vi "Receive Shortcut Menu Selection Event.vi"(8 "error in (no error)":errorcluster, 10 "ShortcutMenuSelectionMsg":refnum<class "ShortcutMenuSelectionMsg.lvclass">, 11 "File Explorer In":refnum<class "File Explorer.lvclass">) -> (0 "error out":errorcluster, 3 "File Explorer Out":refnum<class "File Explorer.lvclass">)   [LabVIEW 2020, in "File Explorer.lvlib" / "File Explorer.lvclass"]
doc: "<License>\nCopyright © 2017 Composed Systems, LLC | All rights reserved\nwww.composed.io\n\nAuthor: Ethan Stern <ethan.stern@composed.io>\n\nThis software is provided \"AS IS\" WITHOUT WARRANTIES, either express or implied, AND IS FOR EDUCATIONAL PURPOSES ONLY.\n</License>"
uses:
  <vilib>/gpm_packages/@cs/file-explorer-extension/Source/File Explorer/File Explorer/File Explorer.lvclass
  <vilib>/gpm_packages/@cs/mva-viewable/Source/ActorEvents/IEventAggregator Messages/ShortcutMenuSelectionMsg/ShortcutMenuSelectionMsg.lvclass
  <vilib>/gpm_packages/@cs/mva-viewable/Source/ActorEvents/IEventAggregator Messages/ShortcutMenuSelectionMsg/ShortcutMenuSelectionMsg.lvclass/ShortcutMenuSelectionMsg.ctl
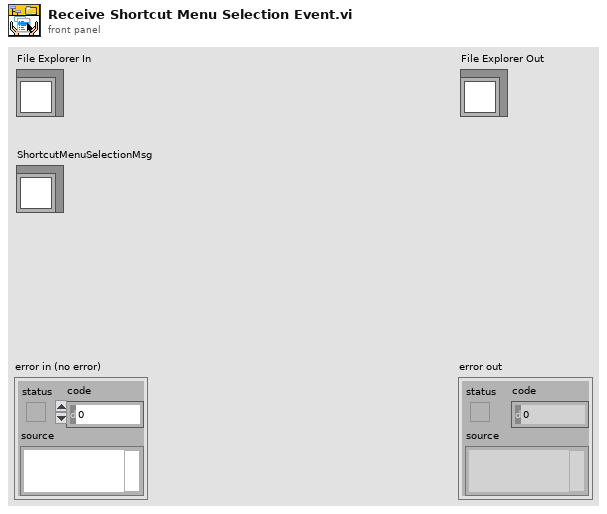
[diagram p1: front panel]
types:
  T1 = typedef "LVPoint32TypeDef.ctl" = cluster{"Horizontal":i32, "Vertical":i32}
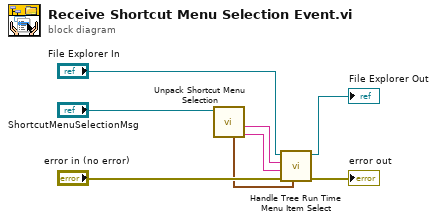
[diagram p0: block diagram]
diagram:
  n1 = call <vilib>:"Unpack Shortcut Menu Selection.vi"("ShortcutMenuSelectionMsg"="ShortcutMenuSelectionMsg") -> ("Item Path"=w6:string, "Item Tag"=w7:string, "Coords"=w1:T1)  [unwired: 3 in, 5 out]
  n2 = call-dynamic "Handle Tree Run Time Menu Item Select.vi"("Coords"=w1, "error in (no error)"="error in (no error)", "ItemPath"=w6, "ItemTag"=w7, "File Explorer in"="File Explorer In") -> ("error out"=→"error out":errorcluster, "File Explorer out"=→"File Explorer Out":refnum<class "File Explorer.lvclass">)  [unwired: 5 in]
